vi "TCP Read.vi"(7 "Timeout (1000 ms )":i32=1000, 8 "Error In":errorcluster, 10 "Bytes To Read":i32=4, 11 "LINX Device Config":T1={"Interface"=enum."TCP", "COM Port"="COM5", "TCP Configuration"={"IP Address"="10.2.106.213", "Port"=6921}, "Device Family"=enum."Digilent", "Device ID"=1, "Device Name"="chipKIT uC32", "TCP Ref"=refnum}) -> (0 "Error Out":errorcluster, 2 "Data":string, 3 "LINX Device Config":T1={"Interface"=enum."TCP", "COM Port"="COM5", "TCP Configuration"={"IP Address"="10.2.106.213", "Port"=6921}, "Device Family"=enum."Digilent", "Device ID"=1, "Device Name"="chipKIT uC32", "TCP Ref"=refnum})   [LabVIEW 2013, in "LVH-LINX.lvlib" / "Device.lvlib"]
uses:
  <vilib>/LabVIEW Hacker/LINX/Private/Device/Device.lvlib
  <vilib>/LabVIEW Hacker/LINX/Private/Device/Type Defs/LINX Device Config.ctl
  <vilib>/LabVIEW Hacker/LINX/Private/Type Defs/Interface.ctl
  <vilib>/LabVIEW Hacker/LINX/Private/Device/Type Defs/TCP Config.ctl
  <vilib>/LabVIEW Hacker/LINX/Private/Type Defs/Device Family.ctl
  <vilib>/LabVIEW Hacker/LINX/LVH-LINX.lvlib
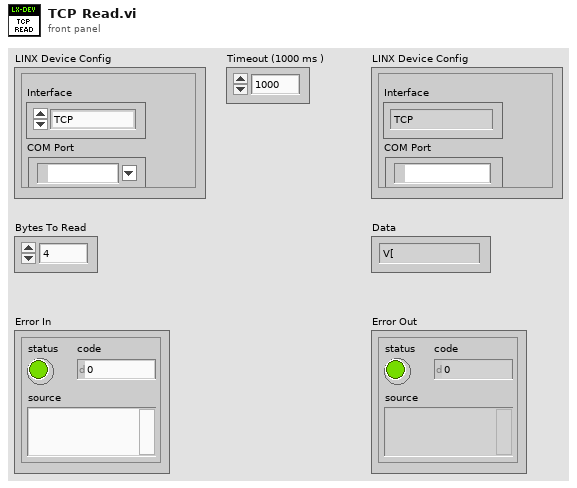
[diagram p1: front panel]
types:
  T1 = typedef "LVH-LINX.lvlib/Device.lvlib/LINX Device Config.ctl" = cluster{"Interface":T2, "COM Port":refnum<visa-resource-name>, "TCP Configuration":T3, "Device Family":T4, "Device ID":u8, "Device Name":string, "TCP Ref":refnum<k5>}
  T2 = typedef "LVH-LINX.lvlib/Interface.ctl" = enum16{"Serial", "TCP"}
  T3 = typedef "LVH-LINX.lvlib/Device.lvlib/TCP Config.ctl" = cluster{"IP Address":string, "Port":u16}
  T4 = typedef "LVH-LINX.lvlib/Device Family.ctl" = enum8{"National Instruments", "Digilent", "Arduino"}
  T5 = enum16{"Standard", "Buffered", "CRLF", "Immediate"}
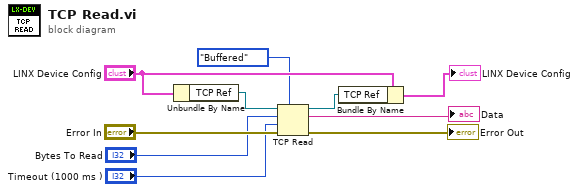
[diagram p0: block diagram]
diagram:
  n1 = Unbundle By Name("LINX Device Config") -> ("TCP Ref"=w5:refnum<k5>)
  n2 = TCP Read(connection ID=w5, bytes to read="Bytes To Read", error in (no error)="Error In", 7:T5."Buffered" ("mode (standard)"), 9:"Timeout (1000 ms )") -> (connection ID out=w8:refnum<k5>, data out=→"Data":string, error out=→"Error Out":errorcluster)
  n3 = Bundle By Name(cluster="LINX Device Config", "TCP Ref"=w8) -> (→"LINX Device Config":T1)
